vi "computeIRFAlignment.vi"(8 "error in (no error)":errorcluster, 10 "fIRF temp":dbl[](array[numeric]), 11 "LaguerreDeconEngineClass in":refnum<class "LaguerreDeconEngineClass.lvclass">) -> (0 "error out":errorcluster, 2 "iRF shift":dbl, 3 "LaguerreDeconEngineClass out":refnum<class "LaguerreDeconEngineClass.lvclass">)   [LabVIEW 2020, in "LaguerreDeconEngineClass.lvclass"]
uses:
  LaguerreDeconEngineClass.lvclass
  LaguerreDeconEngineClass.lvclass/LaguerreDeconEngineClass.ctl
panel:
  out "SSE Graph":cluster{dbl[], dbl[]}(graph)
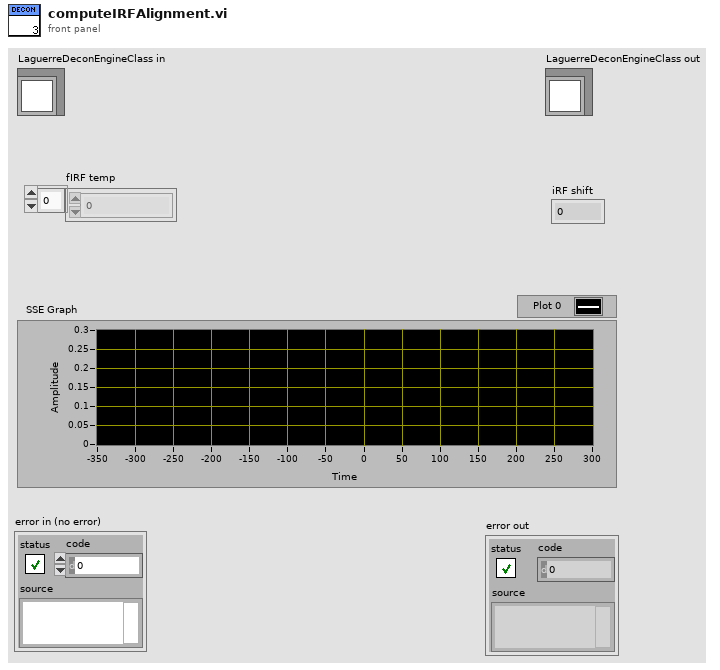
[diagram p1: front panel]
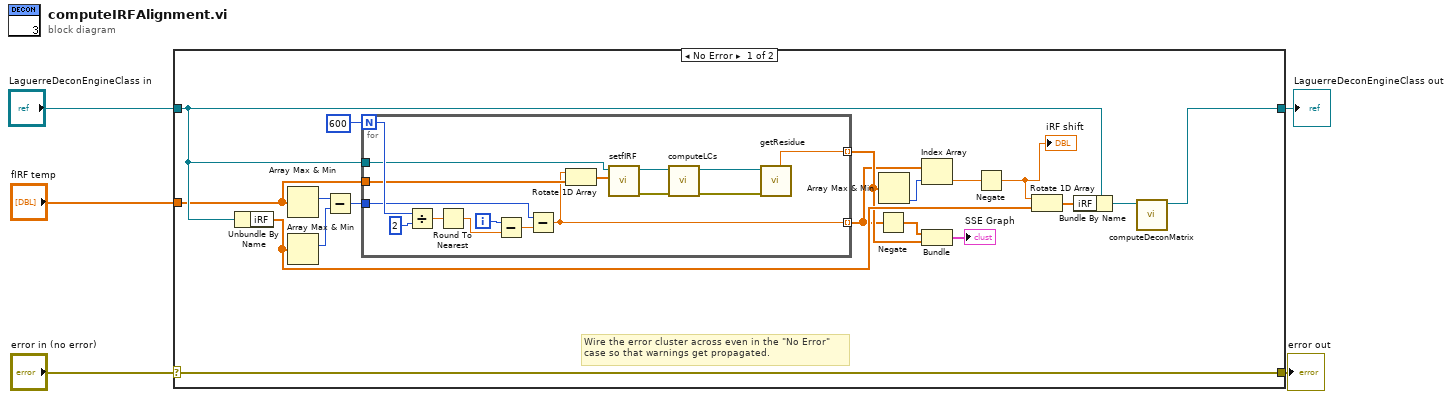
[diagram p0: block diagram]
diagram:
  n1 = case shown="No Error" "error in (no error)" {
    selector: "error in (no error)" -> [w23 w41]
    tunnel: [w23 w41] -> w4
    tunnel: [w7 w40] -> w2
    tunnel: "LaguerreDeconEngineClass in" -> [w17 w40]
    tunnel: "fIRF temp" -> [w9 _]
    frame No Error {
      # "Wire the error cluster across even in the \"No Error\"\ncase so that warnings get propagated."
      n2 = Unbundle By Name(w17) -> ("iRF"=w16:dbl[])
      n3 = Array Max & Min(array=w9) -> (max index (indices)=w21:i32)  [unwired: 3 out]
      n4 = Array Max & Min(array=w16) -> (max index (indices)=w22:i32)  [unwired: 3 out]
      n5 = Subtract(x=w21, y=w22) -> (x-y=w19:i32)
      n6 = for {
        N: 600 -> [w38]
        tunnel: w19 -> [w34]
        tunnel: w9 -> [w33]
        tunnel: w17 -> [w32]
        tunnel: [w26] -> w13 mode=indexing
        tunnel: [w25] -> w10 mode=indexing
        i -> [w39]
        n7 = Divide(x=w38, y=2) -> (x/y=w36:dbl)
        n8 = Round To Nearest(number=w36) -> (nearest integer value=w35:dbl)
        n9 = Subtract(x=w39, y=w35) -> (x-y=w24:dbl)
        n10 = Subtract(x=w34, y=w24) -> (x-y=w25:dbl)
        n11 = Rotate 1D Array(1:w33, 2:w25) -> (0:w31:dbl[])
        n12 = call "setfIRF.vi"("fIRF"=w31, "LaguerreDeconEngineClass in"=w32) -> ("error out"=w30:errorcluster, "LaguerreDeconEngineClass out"=w29:refnum<class "LaguerreDeconEngineClass.lvclass">)  [unwired: 8 in]
        n13 = call "computeLCs.vi"("error in (no error)"=w30, "LaguerreDeconClass in"=w29) -> ("error out"=w27:errorcluster, "LaguerreDeconClass out"=w28:refnum<class "LaguerreDeconEngineClass.lvclass">)  [unwired: 8 in]
        n14 = call "getResidue.vi"("error in (no error)"=w27, "LaguerreDeconEngineClass in"=w28) -> ("SSE"=w26:dbl)  [unwired: 5 in, 4 out]
      }
      n15 = Negate(x=w10) -> (-x=w11:dbl[])
      n16 = Array Max & Min(array=w13) -> (min index (indices)=w18:i32)  [unwired: 3 out]
      n17 = Index Array(array=w10, index=w18) -> (element=w15:dbl)
      n18 = Bundle(w11, w13) -> (→"SSE Graph":cluster{dbl[], dbl[]})  [unwired: 1 in]
      n19 = Negate(x=w15) -> (-x=w6:dbl)
      "iRF shift" <- w6
      n20 = Rotate 1D Array(1:w16, 2:w6) -> (0:w14:dbl[])
      n21 = Bundle By Name(cluster=w17, "iRF"=w14) -> (w8:refnum<class "LaguerreDeconEngineClass.lvclass">)
      n22 = call "computeDeconMatrix.vi"("LaguerreDeconClass in"=w8) -> ("LaguerreDeconClass out"=w7:refnum<class "LaguerreDeconEngineClass.lvclass">)  [unwired: 9 in, 1 out]
    }
    frame Error {
    }
  }
  "error out" <- w4
  "LaguerreDeconEngineClass out" <- w2
